vi "Open Line Interlock Configuration.vi"(8 "error in (no error)":errorcluster, 9 "Manual Mode (False)":bool, 10 "Sample Line (All Closed)":T1, 11 "Sample Line in":refnum<class "Sample Line.lvclass">) -> (0 "error out":errorcluster, 1 "Interlock Chain":refnum<class "Interlock Chain.lvclass">, 2 "Sample Line out":T1, 3 "Sample Line out":refnum<class "Sample Line.lvclass">)   [LabVIEW 2015, in "cRIO-Carbondioxide.lvlib" / "CO2-Actor.lvlib" / "Sample Line.lvclass"]
uses:
  Sample Line.lvclass
  Interlocks/Interlock Chain/Interlock Chain.lvclass
  Controls/Sample Line State Enumerator.ctl
  Interlocks/Controls/Add IL to -Enumerator.ctl
  Interlocks/Interlock/Interlock.lvclass
  Interlocks/Interlock Sample/Interlock Sample.lvclass
  Interlocks/Interlock Sample/Action Enum.ctl
  subs/Sample/Sample.lvclass
  Interlocks/Interlock I32/Pass/IL I32 Pass.lvclass
  Interlocks/Interlock I32/Pass/IL I32 Pass.lvclass/IL I32 Pass.ctl
  Transfer Line/Transfer Line.lvclass
  CO2 Actor Messages/Ping Msg/Ping Msg.lvclass/Ping Msg.ctl
  <vilib>/ActorFramework/Message Enqueuer/Message Enqueuer.lvclass/Message Enqueuer.ctl
  Transfer Line/Transfer Line.lvclass/Transfer Line.ctl
  Interlocks/Interlock Chain/Interlock Chain.lvclass/Interlock Chain.ctl
  <vilib>/ActorFramework/Message Enqueuer/Enqueue.vi
  <vilib>/ActorFramework/Message Priority Queue/Priority Enqueue.vi
  subs/Sample/Read Sample From Container.vi
  CO2 Actor Messages/Ping Msg/Ping Msg.lvclass
  <vilib>/ActorFramework/Actor/Actor.lvclass
  CO2 Actor/CO2 Actor.lvclass
  cRIO-CO2/cRIO-CO2.lvclass
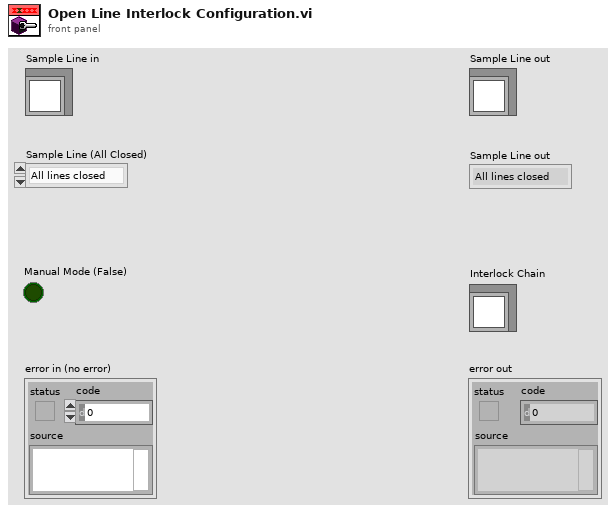
[diagram p1: front panel]
types:
  T1 = typedef "Sample Line State Enumerator.ctl" = enum16{"All lines closed", "Sample line 1.", "Sample line 2.", "Sample line 3.", "Sample line 4.", "Sample line 5.", "Out of range"}
  T2 = typedef "Add IL to -Enumerator.ctl" = enum16{"Deny", "Allow", "None"}
  T3 = typedef "Action Enum.ctl" = enum16{"Allow", "Deny"}
  T4 = typedef "Sample Container.ctl" = cluster{"Sample In":refnum<k21>, "Sample Name":refnum<k21>, "Ti Cathode":refnum<k21>, "SampleQ":refnum<queue>}
  T5 = typedef "Dedicated Enqueuers.ctl" = cluster{"Freezers":cluster{"Syringe":refnum<class "Message Enqueuer.lvclass">, "Tank 1":refnum<class "Message Enqueuer.lvclass">, "Tank 2":refnum<class "Message Enqueuer.lvclass">, "Tank 3":refnum<class "Message Enqueuer.lvclass">, "Tank 4":refnum<class "Message Enqueuer.lvclass">}, "Heaters":cluster{"Syringe":refnum<class "Message Enqueuer.lvclass">, "Piston":refnum<class "Message Enqueuer.lvclass">}, "Blowers":cluster{"Tank 1":refnum<class "Message Enqueuer.lvclass">, "Tank 2":refnum<class "Message Enqueuer.lvclass">, "Tank 3":refnum<class "Message Enqueuer.lvclass">, "Tank 4":refnum<class "Message Enqueuer.lvclass">, "Syringe":refnum<class "Message Enqueuer.lvclass">}, "Sample Line":refnum<class "Message Enqueuer.lvclass">, "Storage Line":refnum<class "Message Enqueuer.lvclass">, "Transfer Line":refnum<class "Message Enqueuer.lvclass">, "Syringe Stepper":refnum<class "Message Enqueuer.lvclass">, "Syringe Line":refnum<class "Message Enqueuer.lvclass">, "Capillary Line":refnum<class "Message Enqueuer.lvclass">, "Preparation Line":refnum<class "Message Enqueuer.lvclass">, "Turbo":refnum<class "Message Enqueuer.lvclass">, "Vacuum":refnum<class "Message Enqueuer.lvclass">, "He Line":refnum<class "Message Enqueuer.lvclass">, "Cylinder":refnum<class "Message Enqueuer.lvclass">}
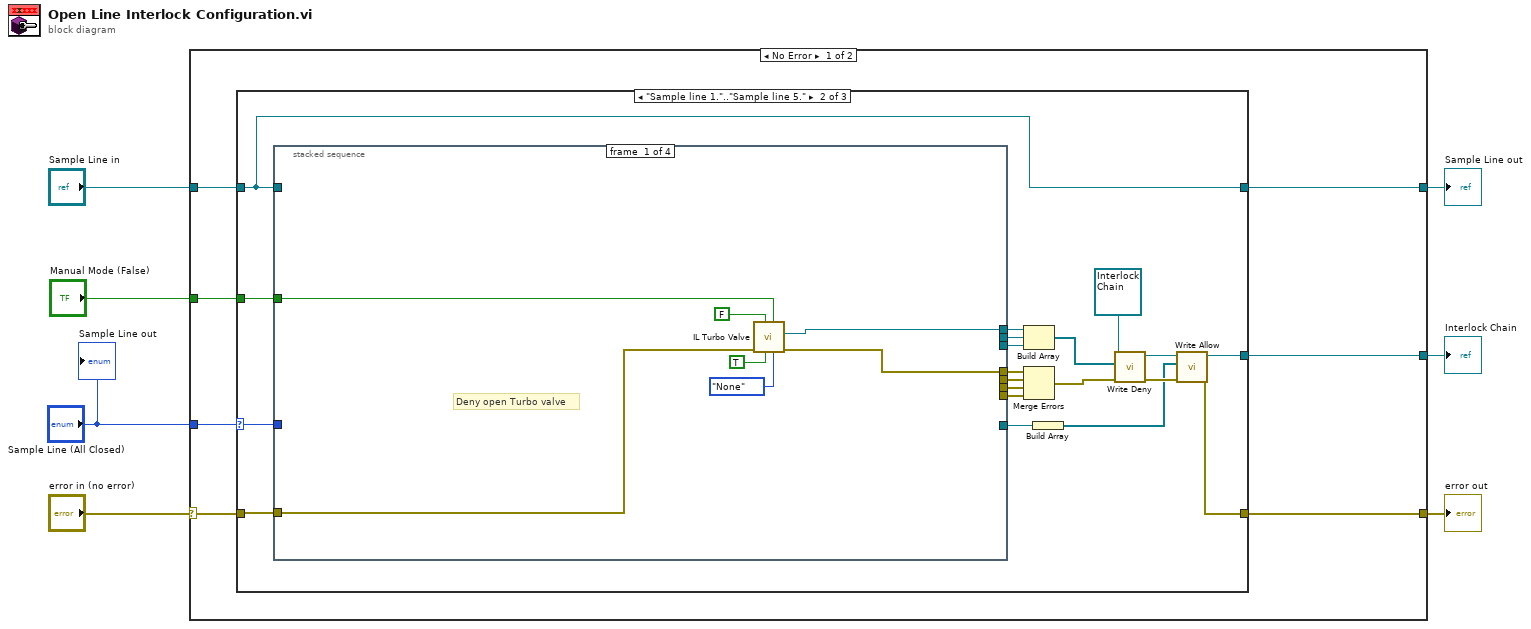
[diagram p0: block diagram]
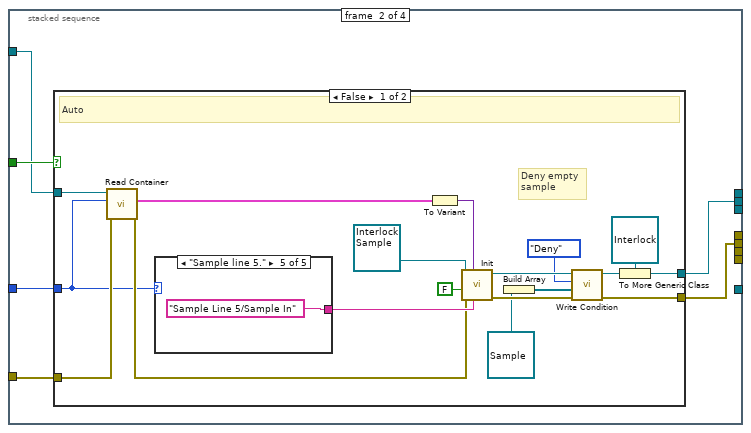
[diagram p3: hidden frame]
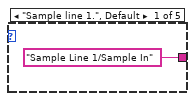
[diagram p4: hidden frame]
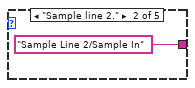
[diagram p5: hidden frame]
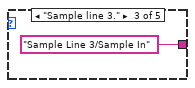
[diagram p6: hidden frame]
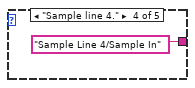
[diagram p7: hidden frame]
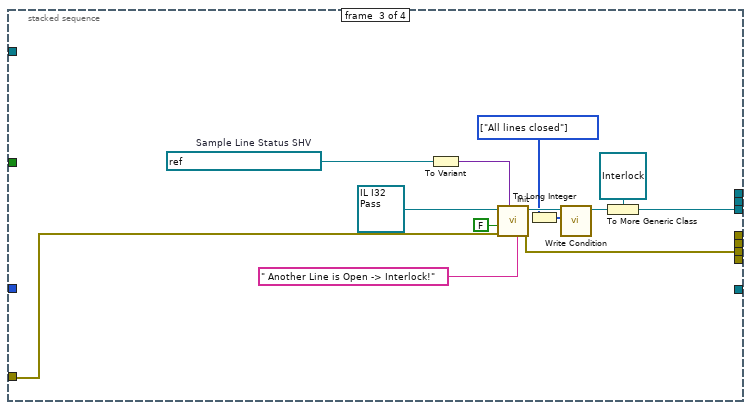
[diagram p9: hidden frame]
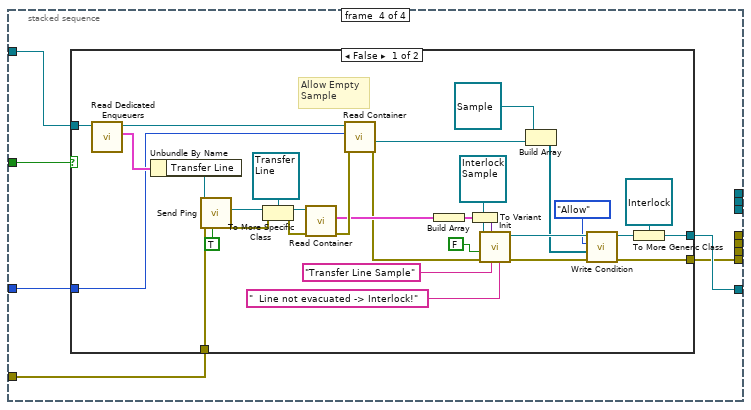
[diagram p10: hidden frame]
diagram:
  n1 = case shown="No Error" "error in (no error)" {
    selector: "error in (no error)" -> [w14 w128]
    tunnel: [w10 w128] -> w6
    tunnel: [w9 w127] -> w4
    tunnel: "Sample Line in" -> [w11 w127]
    tunnel: [w13 _] -> w3
    tunnel: "Sample Line (All Closed)" -> [w12 _]
    tunnel: "Manual Mode (False)" -> [w8 _]
    frame No Error {
      n2 = case shown="\"Sample line 1.\"..\"Sample line 5.\"" w12 {
        selector: w12 -> [_ w33 _]
        tunnel: w14 -> [w16 w34 w126]
        tunnel: [w16 w23 w126] -> w10
        tunnel: [_ w25 _] -> w13
        tunnel: w11 -> [w15 w22 w125]
        tunnel: [w15 w22 w125] -> w9
        tunnel: w8 -> [_ w17 _]
        frame "All lines closed", Default {
          # "No interlock"
          # "Close all lines. No Interlock chain."
        }
        frame "Sample line 1.".."Sample line 5." {
          n3 = stacked-sequence {
            tunnel: [w43 _ _ _] -> w36
            tunnel: [w42 _ _ _] -> w35
            tunnel: w34 -> [w41 w49 w84 w91]
            tunnel: w33 -> [_ w46 _ w88]
            tunnel: [_ w48 _ _] -> w32
            tunnel: [_ w47 _ _] -> w31
            tunnel: [_ _ w86 _] -> w30
            tunnel: [_ _ w85 _] -> w29
            tunnel: [_ _ _ w92] -> w18
            tunnel: w22 -> [_ w44 _ w90]
            tunnel: [_ _ _ w89] -> w21
            tunnel: w17 -> [w40 w45 _ w87]
            frame #0 {
              # "Deny open Turbo valve"
              n4 = call "IL Turbo Valve.vi"("Add to (Deny)"=Add_IL_to_-Enumerator."None", "Ignore (F)"=w40, "Interlock Condition (ON/OFF)"=TRUE, "Stop Self on IL? (T)"=FALSE, "error in (no error)"=w41) -> ("error out"=w42:errorcluster, "IL Turbo Valve"=w43:refnum<class "Interlock.lvclass">)  [unwired: 4 in, 1 out]
            }
            frame #1 {
              n5 = case shown="False" w45 {
                tunnel: w44 -> [w65 _]
                tunnel: w49 -> [w64 w73]
                tunnel: [w58 w73] -> w48
                tunnel: [w54 _] -> w47
                tunnel: w46 -> [w52 _]
                frame False {
                  # "Deny empty\nsample"
                  # "Auto"
                  n6 = call "Read Container.vi"("error in (no error)"=w64, "Sample Line (All Closed)"=w52, "Sample Line in"=w65) -> ("error out"=w63:errorcluster, "Containers"=w51:T4[])  [unwired: 5 in, 2 out]
                  n7 = case shown="\"Sample line 5.\"" w52 {
                    tunnel: ["Sample Line 1/Sample In" ("Name (SHV Name if empty)") "Sample Line 2/Sample In" ("Name (SHV Name if empty)") "Sample Line 3/Sample In" ("Name (SHV Name if empty)") "Sample Line 4/Sample In" ("Name (SHV Name if empty)") "Sample Line 5/Sample In" ("Name (SHV Name if empty)")] -> w66
                    frame "Sample line 1.", Default {
                    }
                    frame "Sample line 2." {
                    }
                    frame "Sample line 3." {
                    }
                    frame "Sample line 4." {
                    }
                    frame "Sample line 5." {
                    }
                  }
                  n8 = To Variant(anything=w51) -> (Variant=w56:variant)
                  n9 = call-dynamic "Init.vi"("Name (SHV Name if empty)"=w66, "Sample Containers SHV (Array!)"=w56, "error in (no error)"=w63, "Stop Self on IL? (T)"=FALSE, "Interlock Sample in"=refnum<class "Interlock Sample.lvclass"> refnum ("Interlock Sample.lvclass")) -> ("error out"=w59:errorcluster, "Interlock Sample out"=w61:refnum<class "Interlock Sample.lvclass">)  [unwired: 5 in]
                  n10 = Build Array(refnum<class "Sample.lvclass"> refnum ("Sample.lvclass")) -> (w53:refnum<class "Sample.lvclass">[])
                  n11 = call "Write Condition.vi"("error in (no error)"=w59, "Samples"=w53, "Action (Allow)"=Action_Enum."Deny", "Interlock Sample in"=w61) -> ("error out"=w58:errorcluster, "Interlock Sample out"=w60:refnum<class "Interlock Sample.lvclass">)  [unwired: 6 in]
                  n12 = To More Generic Class(target class=refnum<class "Interlock.lvclass"> refnum ("Interlock.lvclass"), reference=w60) -> (generic class reference=w54:refnum<class "Interlock.lvclass">)
                }
                frame True {
                  # "Manual"
                }
              }
            }
            frame #2 {
              w77 = T1[] [enum."All lines closed"] items=["All lines closed", "Sample line 1.", "Sample line 2.", "Sample line 3.", "Sample line 4.", "Sample line 5.", "Out of range"] ("Deny")
              w80 = refnum<k21> "ni.var.psp://10.2.0.20/AMS Gas SHV/Sample Lines/Sample Line Status"  # Sample Line Status SHV
              n13 = To Variant(anything=w80) -> (Variant=w75:variant)
              n14 = call-dynamic "Init.vi"("Interlock message (\" -> Interlock!\")"=" Another Line is Open -> Interlock!" ("Interlock message (\" -> Interlock!\")"), "SHV"=w75, "error in (no error)"=w84, "Stop Self on IL? (T)"=FALSE, "Interlock in"=refnum<class "IL I32 Pass.lvclass"> refnum ("Interlock Allow.lvclass")) -> ("error out"=w85:errorcluster, "Interlock out"=w83:refnum<class "IL I32 Pass.lvclass">)  [unwired: 5 in]
              n15 = To Long Integer(number=w77) -> (32bit integer=w78:i32[])
              n16 = call "Write Condition.vi"("Allow"=w78, "Interlock I32 in"=w83) -> ("Interlock I32 out"=w81:refnum<class "IL I32 Pass.lvclass">)  [unwired: 9 in]
              n17 = To More Generic Class(target class=refnum<class "Interlock.lvclass"> refnum ("Interlock.lvclass"), reference=w81) -> (generic class reference=w86:refnum<class "Interlock.lvclass">)
            }
            frame #3 {
              n18 = case shown="False" w87 {
                tunnel: [w118 _] -> w92
                tunnel: w91 -> [w110 w124]
                tunnel: w90 -> [w108 _]
                tunnel: [w105 w124] -> w89
                tunnel: w88 -> [w97 _]
                frame False {
                  # "Allow Empty\nSample"
                  n19 = call "Read Dedicated Enqueuers.vi"("CO2 Actor in"=w108) -> ("Dedicated Enqueuers"=w98:T5, "CO2 Actor out"=w107:refnum<class "Sample Line.lvclass">)  [unwired: 7 in, 2 out]
                  n20 = Unbundle By Name(w98) -> ("Transfer Line"=w111:refnum<class "Message Enqueuer.lvclass">)
                  n21 = call "Send Ping.vi"("Return Self (F)"=TRUE, "error in (no error)"=w110, "Message Enqueuer"=w111) -> ("error out"=w112:errorcluster, "Actor out"=w116:refnum<class "Actor.lvclass">)  [unwired: 5 in, 2 out]
                  n22 = To More Specific Class(target class=refnum<class "Transfer Line.lvclass"> refnum ("Transfer Line in"), reference=w116, error in=w112) -> (specific class reference=w114:refnum<class "Transfer Line.lvclass">, error out=w113:errorcluster)
                  n23 = call "Read Container.vi"("error in (no error)"=w113, "Transfer Line in"=w114) -> ("error out"=w109:errorcluster, "Sample Container"=w106:T4)  [unwired: 5 in, 3 out]
                  n24 = call "Read Container.vi"("error in (no error)"=w109, "Sample Line (All Closed)"=w97, "Sample Line in"=w107) -> ("error out"=w95:errorcluster, "Sample"=w94:refnum<class "Sample.lvclass">)  [unwired: 5 in, 2 out]
                  n25 = Build Array(w106) -> (w96:T4[])
                  n26 = To Variant(anything=w96) -> (Variant=w100:variant)
                  n27 = call-dynamic "Init.vi"("Interlock message (\" -> Interlock!\")"="  Line not evacuated -> Interlock!" ("Interlock message (\" -> Interlock!\")"), "Name (SHV Name if empty)"="Transfer Line Sample", "Sample Containers SHV (Array!)"=w100, "error in (no error)"=w95, "Stop Self on IL? (T)"=FALSE, "Interlock Sample in"=refnum<class "Interlock Sample.lvclass"> refnum ("Interlock Sample.lvclass")) -> ("error out"=w122:errorcluster, "Interlock Sample out"=w121:refnum<class "Interlock Sample.lvclass">)  [unwired: 4 in]
                  n28 = Build Array(refnum<class "Sample.lvclass"> refnum ("element"), w94) -> (w103:refnum<class "Sample.lvclass">[])
                  n29 = call "Write Condition.vi"("error in (no error)"=w122, "Samples"=w103, "Action (Allow)"=Action_Enum."Allow", "Interlock Sample in"=w121) -> ("error out"=w105:errorcluster, "Interlock Sample out"=w119:refnum<class "Interlock Sample.lvclass">)  [unwired: 6 in]
                  n30 = To More Generic Class(target class=refnum<class "Interlock.lvclass"> refnum ("Interlock.lvclass"), reference=w119) -> (generic class reference=w118:refnum<class "Interlock.lvclass">)
                }
                frame True {
                }
              }
            }
          }
          n31 = Build Array(w36, w31, w30) -> (w27:refnum<class "Interlock.lvclass">[])
          n32 = Merge Errors(w35, w32, w29, w21) -> (w20:errorcluster)
          n33 = Build Array(w18) -> (w19:refnum<class "Interlock.lvclass">[])
          n34 = call "Write Deny.vi"("error in (no error)"=w20, "Deny"=w27, "Interlock Chain in"=refnum<class "Interlock Chain.lvclass"> refnum) -> ("error out"=w24:errorcluster, "Interlock Chain out"=w26:refnum<class "Interlock Chain.lvclass">)  [unwired: 7 in]
          n35 = call "Write Allow.vi"("error in (no error)"=w24, "Allow"=w19, "Interlock Chain in"=w26) -> ("error out"=w23:errorcluster, "Interlock Chain out"=w25:refnum<class "Interlock Chain.lvclass">)  [unwired: 7 in]
        }
        frame "Out of range" {
          # "No Interlock Chain. \nLet the Sample Line Actor deside\nwhat to do"
          # "Out of range."
        }
      }
    }
    frame Error {
    }
  }
  "error out" <- w6
  "Sample Line out" <- w4
  "Interlock Chain" <- w3
  "Sample Line out" <- "Sample Line (All Closed)"
